vi "Bar Code Reader.vi"() -> ()   [LabVIEW 2016]
uses:
  <vilib>/NXT/Dual Mode Library/Sensors/EV3_Color_Color.vi
  <vilib>/NXT/NXTIO Xnodes/NXTIONodeSubVIs/LEGOMoveAllMotors.vi
  <vilib>/NXT/NXTIO Xnodes/NXTIONodeSubVIs/LEGOMoveAllMotorsDistance.vi
  <vilib>/NXT/Dual Mode Library/Waits/Wait_Num.vi
  <vilib>/NXT/Block Support/NXT_OutputPort.ctl
  <vilib>/NXT/Subs/LVHSConnector.ctl
  <vilib>/NXT/NXTIO Xnodes/NXTIOXNode/NXTIO.xnode
  <vilib>/NXT/LegoClasses/BrickReference/BrickReference.lvclass
panel:
  out "Type 2":dbl
  out "Type 1":dbl
  out "Material 4":string
  out "Type 2":dbl
  out "Type 1":dbl
  out "Material 3":string
  out "Type 2":dbl
  out "Type 1":dbl
  out "Material 2":string
  out "Type 2":dbl
  out "Type 1":dbl
  out "String 3":string
  out "String 2":string
  out "Material":string
  out "String":string
  out "Numeric":dbl
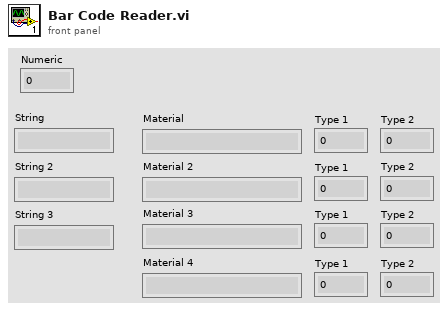
[diagram p1: front panel]
types:
  T1 = typedef "ColorSensorColors.ctl" = enum16{"No Color", "Black", "Blue", "Green", "Yellow", "Red", "White", "Brown"}
  T2 = typedef "LVHSConnector.ctl" = refnum<class "BrickReference.lvclass">
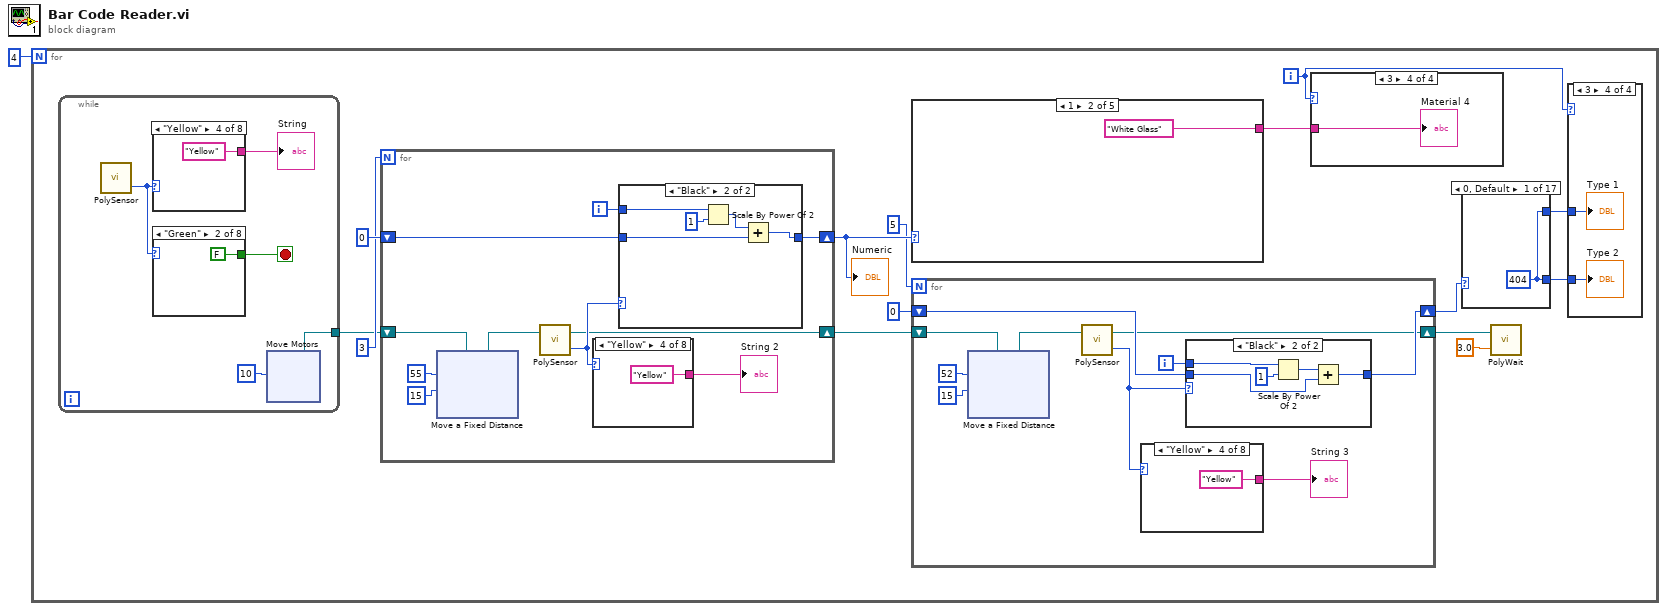
[diagram p0: block diagram]
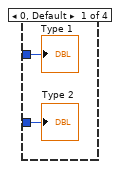
[diagram p2: hidden frame]
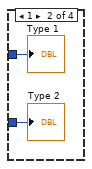
[diagram p3: hidden frame]
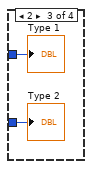
[diagram p4: hidden frame]
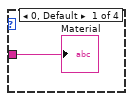
[diagram p5: hidden frame]
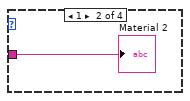
[diagram p6: hidden frame]
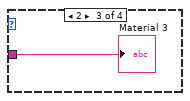
[diagram p7: hidden frame]
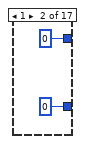
[diagram p8: hidden frame]
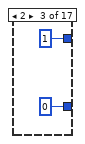
[diagram p9: hidden frame]
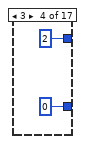
[diagram p10: hidden frame]
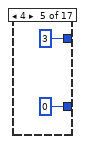
[diagram p11: hidden frame]
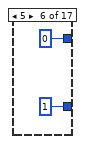
[diagram p12: hidden frame]
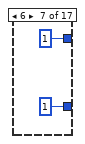
[diagram p13: hidden frame]
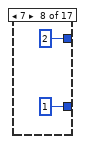
[diagram p14: hidden frame]
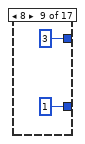
[diagram p15: hidden frame]
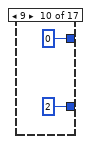
[diagram p16: hidden frame]
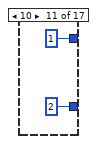
[diagram p17: hidden frame]
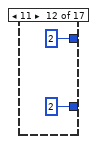
[diagram p18: hidden frame]
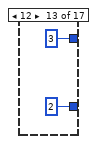
[diagram p19: hidden frame]
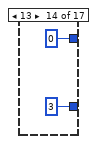
[diagram p20: hidden frame]
diagram:
  n1 = for {
    N: 4 -> [_]
    i -> [w4]
    n2 = while {
      tunnel: [w97] -> w13
      stop <- w101 stop-if-true
      n3 = call-poly <vilib>:"PolySensor.vi"() -> ("Detected Color"=w99:T1)  [unwired: 3 in, 1 out]
      n4 = case shown="\"Yellow\"" w99 {
        tunnel: ["No Color" "Blue" "Green" "Yellow" "Red" "White" "Brown" "Black"] -> w100
        frame "No Color", Default {
        }
        frame "Blue" {
        }
        frame "Green" {
        }
        frame "Yellow" {
        }
        frame "Red" {
        }
        frame "White" {
        }
        frame "Brown" {
        }
        frame "Black" {
        }
      }
      "String" <- w100
      n5 = case shown="\"Green\"" w99 {
        tunnel: [FALSE FALSE FALSE FALSE FALSE FALSE FALSE TRUE] -> w101
        frame "No Color", Default {
        }
        frame "Green" {
        }
        frame "Yellow" {
        }
        frame "Red" {
        }
        frame "White" {
        }
        frame "Brown" {
        }
        frame "Blue" {
        }
        frame "Black" {
        }
      }
      n6 = xnode "Move Motors"("Power/Speed 1"=i8 10) -> ("NXT/EV3"=w97:T2)  [unwired: 2 in]
    }
    n7 = for {
      N: 3 -> [_]
      shift-right: [w134] -> w12
      shift-left: 0 -> [w133]
      shift-right: [w129] -> w8
      shift-left: w13 -> [w126]
      i -> [w130]
      n8 = xnode "Move a Fixed Distance"("Speed 1"=i8 15, "Distance 1"=55, "NXT/EV3"=w126) -> ("NXT/EV3"=w125:T2)  [unwired: 1 in]
      n9 = call-poly <vilib>:"PolySensor.vi"("NXT/EV3"=w125) -> ("Detected Color"=w131:T1, "NXT/EV3"=w129:T2)  [unwired: 2 in]
      n10 = case shown="\"Yellow\"" w131 {
        tunnel: ["No Color" "Blue" "Green" "Yellow" "Red" "White" "Brown" "Black"] -> w132
        frame "No Color", Default {
        }
        frame "Blue" {
        }
        frame "Green" {
        }
        frame "Yellow" {
        }
        frame "Red" {
        }
        frame "White" {
        }
        frame "Brown" {
        }
        frame "Black" {
        }
      }
      "String 2" <- w132
      n11 = case shown="\"Black\"" w131 {
        tunnel: w130 -> [_ w154]
        tunnel: [w150 w152] -> w134
        tunnel: w133 -> [w150 w151]
        frame "White", Default {
        }
        frame "Black" {
          n12 = Scale By Power Of 2(n=w154, x=1) -> (x*2^n=w153:i32)
          n13 = Add(x=w153, y=w151) -> (x+y=w152:i32)
        }
      }
    }
    "Numeric" <- w12
    n14 = case shown="1" w12 {
      tunnel: ["Something has gone wrong" "White Glass" "Red Glass" "Blue Glass" "Steel/HDPE"] -> w11
      frame 0, Default {
      }
      frame 1 {
      }
      frame 2 {
      }
      frame 3 {
      }
      frame 4 {
      }
    }
    n15 = for {
      N: 5 -> [_]
      shift-right: [w70] -> w7
      shift-left: 0 -> [w69]
      shift-right: [w65] -> w3
      shift-left: w8 -> [w62]
      i -> [w66]
      n16 = xnode "Move a Fixed Distance"("Speed 1"=i8 15, "Distance 1"=52, "NXT/EV3"=w62) -> ("NXT/EV3"=w61:T2)  [unwired: 1 in]
      n17 = call-poly <vilib>:"PolySensor.vi"("NXT/EV3"=w61) -> ("Detected Color"=w67:T1, "NXT/EV3"=w65:T2)  [unwired: 2 in]
      n18 = case shown="\"Yellow\"" w67 {
        tunnel: ["No Color" "Blue" "Green" "Yellow" "Red" "White" "Brown" "Black"] -> w68
        frame "No Color", Default {
        }
        frame "Blue" {
        }
        frame "Green" {
        }
        frame "Yellow" {
        }
        frame "Red" {
        }
        frame "White" {
        }
        frame "Brown" {
        }
        frame "Black" {
        }
      }
      "String 3" <- w68
      n19 = case shown="\"Black\"" w67 {
        tunnel: w66 -> [_ w90]
        tunnel: [w86 w88] -> w70
        tunnel: w69 -> [w86 w87]
        frame "White", Default {
        }
        frame "Black" {
          n20 = Scale By Power Of 2(n=w90, x=1) -> (x*2^n=w89:i32)
          n21 = Add(x=w89, y=w87) -> (x+y=w88:i32)
        }
      }
    }
    n22 = case shown="3" w4 {
      tunnel: w11 -> [w24 w25 w26 w27]
      frame 0, Default {
        "Material" <- w24
      }
      frame 1 {
        "Material 2" <- w25
      }
      frame 2 {
        "Material 3" <- w26
      }
      frame 3 {
        "Material 4" <- w27
      }
    }
    n23 = case shown="0, Default" w7 {
      tunnel: [w28 0 1 2 3 0 1 2 3 0 1 2 3 0 1 2 3] -> w6
      tunnel: [w28 0 0 0 0 1 1 1 1 2 2 2 2 3 3 3 3] -> w5
      frame 0, Default {
        w28 = 404
      }
      frame 1 {
      }
      frame 2 {
      }
      frame 3 {
      }
      frame 4 {
      }
      frame 5 {
      }
      frame 6 {
      }
      frame 7 {
      }
      frame 8 {
      }
      frame 9 {
      }
      frame 10 {
      }
      frame 11 {
      }
      frame 12 {
      }
      frame 13 {
      }
      frame 14 {
      }
      frame 15 {
      }
      frame 16 {
      }
    }
    n24 = call-poly <vilib>:"PolyWait.vi"("Time (1 sec)"=sgl 3.0, "NXT/EV3"=w3) -> ()  [unwired: 2 in, 1 out]
    n25 = case shown="3" w4 {
      tunnel: w6 -> [w17 w18 w20 w22]
      tunnel: w5 -> [w16 w19 w21 w23]
      frame 0, Default {
        "Type 2" <- w16
        "Type 1" <- w17
      }
      frame 1 {
        "Type 1" <- w18
        "Type 2" <- w19
      }
      frame 2 {
        "Type 1" <- w20
        "Type 2" <- w21
      }
      frame 3 {
        "Type 1" <- w22
        "Type 2" <- w23
      }
    }
  }
